vi "Moving_Statistic_get.vi"(8 "error in (no error)":errorcluster, 11 "Moving_Statistic in":refnum<class "Moving_Statistic.lvclass">) -> (0 "error out":errorcluster, 2 "output cluster":T1, 3 "Moving_Statistic out":refnum<class "Moving_Statistic.lvclass">)   [LabVIEW 2021, in "Moving_Statistic.lvclass"]
uses:
  Moving_Statistic.lvclass
  Moving_Statistic.lvclass/Moving_Statistic.ctl
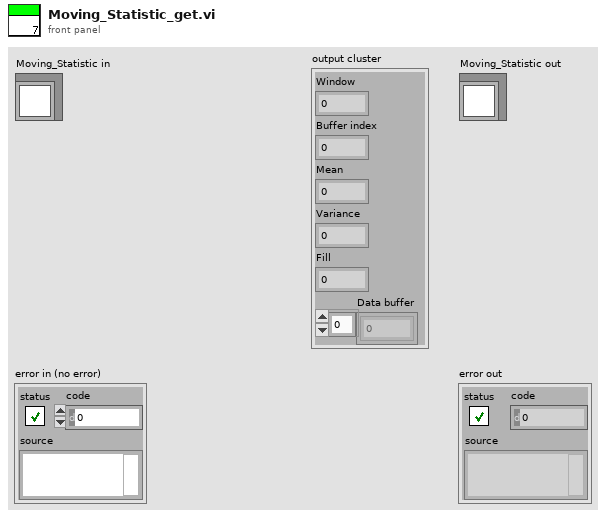
[diagram p1: front panel]
types:
  T1 = cluster{"Window":i32, "Buffer index":i32, "Mean":dbl, "Variance":dbl, "Fill":i32, "Data buffer":dbl[]}
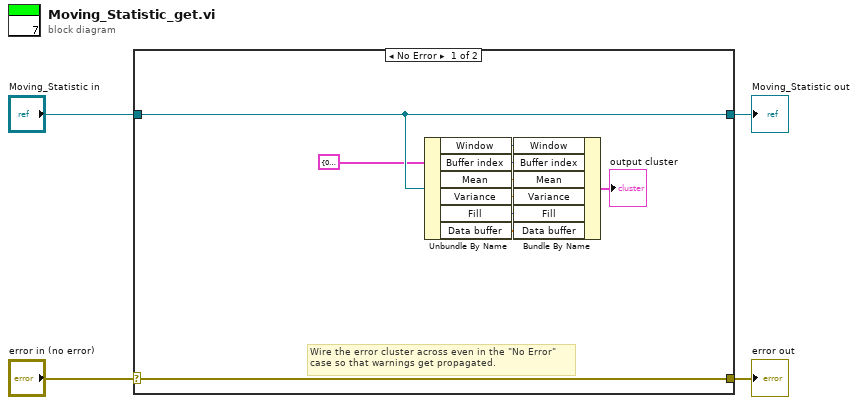
[diagram p0: block diagram]
diagram:
  n1 = case shown="No Error" "error in (no error)" {
    selector: "error in (no error)" -> [w14 w16]
    tunnel: [w14 w16] -> w3
    tunnel: [w13 w15] -> w1
    tunnel: "Moving_Statistic in" -> [w13 w15]
    frame No Error {
      # "Wire the error cluster across even in the \"No Error\"\ncase so that warnings get propagated."
      n2 = Unbundle By Name(w13) -> ("Window"=w12:i32, "Buffer index"=w11:i32, "Mean"=w10:dbl, "Variance"=w9:dbl, "Fill"=w8:i32, "Data buffer"=w7:dbl[])
      n3 = Bundle By Name(cluster=T1 {"Window"=0, "Buffer index"=0, "Mean"=0.0, "Variance"=0.0, "Fill"=0, "Data buffer"=[]} ("input cluster"), "Window"=w12, "Buffer index"=w11, "Mean"=w10, "Variance"=w9, "Fill"=w8, "Data buffer"=w7) -> (→"output cluster":T1)
    }
    frame Error {
    }
  }
  "error out" <- w3
  "Moving_Statistic out" <- w1
